vi "FTW-Ether-CreateServer.vi"(5 "Server Address":string, 7 "Server Identity":string, 11 "error in":errorcluster) -> (4 "Server Endpoint":refnum<class "FTW-Endpoint.lvclass">, 6 "Actual Server Address":string, 8 "Actual Identity":string, 10 "Incoming Requests":refnum<event-registration>, 15 "error out":errorcluster)   [LabVIEW 2013, in "FTW-Actor.lvlib" / "FTW-Ether.lvclass"]
uses:
  FTW-Ether.lvclass
  Endpoint/FTW-Endpoint.lvclass
  Message/Request/FTW-Message-IncomingRequest.lvclass
  FTW-Ether-EndpointType.ctl
panel:
  # "Inputs"
  # "Outputs"
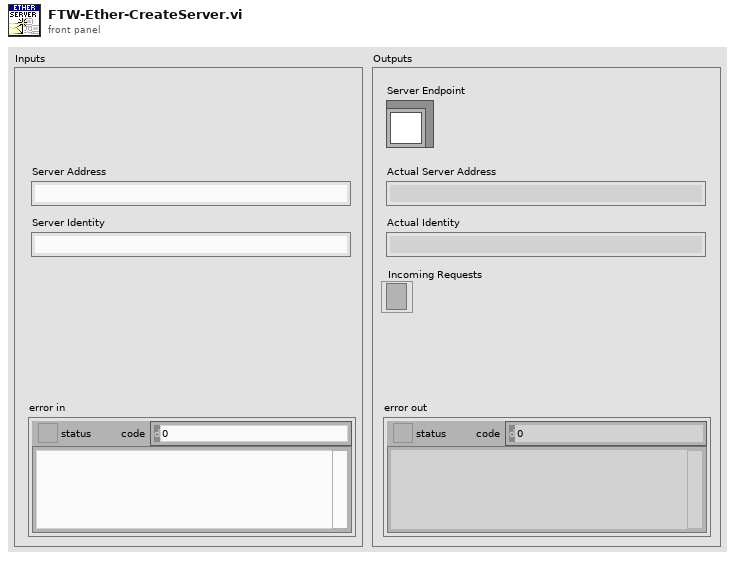
[diagram p1: front panel]
types:
  T1 = typedef "FTW-Actor.lvlib/FTW-Ether.lvclass/FTW-Ether-EndpointType.ctl" = enum16{"Server", "Client", "Publisher", "Subscriber"}
  T2 = typedef "FTW-Actor.lvlib/FTW-Ether.lvclass/FTW-Ether-MessageTransportScheme.ctl" = enum16{"LabVIEW Queues (lvq://)", "LabVIEW Notifiers (lvn://)", "LabVIEW Network Streams (lvns://)"}
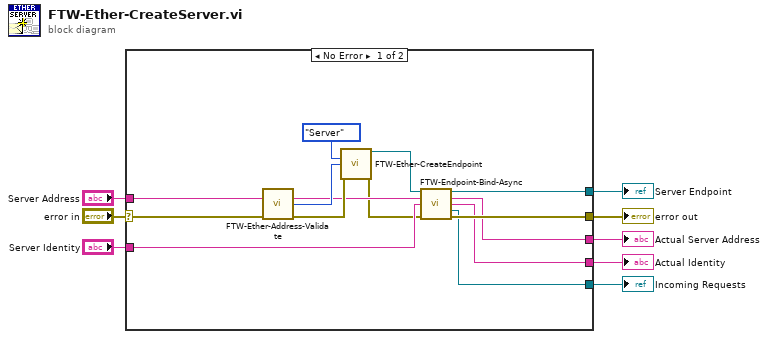
[diagram p0: block diagram]
diagram:
  n1 = case shown="No Error" "error in" {
    selector: "error in" -> [w19 w23]
    tunnel: [w22 _] -> w2
    tunnel: [w21 w23] -> w3
    tunnel: "Server Address" -> [w18 _]
    tunnel: [w15 _] -> w5
    tunnel: "Server Identity" -> [w14 _]
    tunnel: [w13 _] -> w1
    tunnel: [w12 _] -> w4
    frame No Error {
      n2 = call "FTW-Ether-Address-Validate.vi"("Address"=w18, "error in"=w19) -> ("Sanitized Address"=w16:string, "Message Transport Scheme"=w17:T2, "error out"=w20:errorcluster)  [unwired: 11 in]
      n3 = call "FTW-Ether-CreateEndpoint.vi"("Endpoint Type"=FTW-Ether-EndpointType."Server", "Message Transport Scheme"=w17, "error in"=w20) -> ("FTW Endpoint"=w11:refnum<class "FTW-Endpoint.lvclass">, "error out"=w9:errorcluster)  [unwired: 11 in]
      n4 = call-dynamic "FTW-Endpoint-Bind-Async.vi"("FTW Endpoint"=w11, "Endpoint Address"=w16, "Requested Identity"=w14, "error in"=w9) -> ("FTW Endpoint out"=w22:refnum<class "FTW-Endpoint.lvclass">, "Actual Endpoint Address"=w15:string, "Actual Identity"=w12:string, "Incoming Requests"=w13:refnum<event-registration>, "error out"=w21:errorcluster)  [unwired: 7 in]
    }
    frame Error {
    }
  }
  "error out" <- w3
  "Server Endpoint" <- w2
  "Actual Server Address" <- w5
  "Actual Identity" <- w4
  "Incoming Requests" <- w1
